vi "CPP-BLplotter.vi"(0 "Plot Array":cluster{dbl[], dbl[]}[](array[cluster]) {"?" format="%.2f"; "?" format="%.2f"}, 1 "Job Directory":path) -> (2 "Saved Automatically?":bool, 3 "gnuplotScript":string, 4 "Plot data file":path)   [LabVIEW 2014]
uses:
  gnuplotScriptComponents/BLPlottersubVIs/BLTarget.ctl
  gnuplotScriptComponents/BLPlottersubVIs/Resampler.ctl
  gnuplotScriptComponents/at.ctl
  Results_plotter_Global.vi
panel:
  in  "Tab Control":enum32{"Good Shit", "Targets", "Boring Shit"}(tab)
  in  "NormaliseHeight?":bool
  in  "oneshot":bool=TRUE
  in  "U(h)":dbl
  in  "Fit Zmin":dbl=100.0 min=0.0 max=200.0 step=20.0
  in  "autoprint":bool
  out "with d0":cluster{"n":dbl, "d0":dbl, "d0 2":dbl} {"d0 2" format="%#.1e"; "d0" format="%#.1f"; "n" format="%.3f"}
  in  "Fit Zmax":dbl=550.0 min=0.0 max=2000.0 step=50.0
  out "lambda-":dbl format="%_2g"
  out "lambda+":dbl format="%_2g"
  out "lambda(h)":dbl format="%.3g"
  in  "HeightJitter%":dbl min=0.0 max=20.0 step=1.0
  in  "Spectra Folder::":path
  out "Spectrum":cluster{"all rows":dbl[], "all rows":dbl[]}[](graph)
  in  "Stop Button":bool
  in  "Print Button":bool
  out "U,L(U)":cluster{dbl[], dbl[]}[](graph)
  out "TI,Sigma":cluster{dbl[], dbl[]}[](graph)
  in  "MaxFitFreq":dbl
  in  "lambdaSpan(%)":dbl
  in  "integralTweak":dbl=1.0 min=0.8 max=1.2 step=0.01
  out "case":string
  out "No d0":cluster{"n":dbl, "d0":dbl, "d0 2":dbl} {"d0 2" format="%#.1e"; "n" format="%.3f"}
  in  "Spectra?":bool
  in  "Scale":dbl=1.0 min=1.0 max=10000.0 step=50.0
  in  "Zref":dbl=508.0 min=0.0 step=25.0
  in  "BL Scratchpad":T1[](array[typedef]) {"n" min=0.02 max=0.5 step=0.01 format="%.2f"}
  in  "Boundary Layer Targets Folder":path=path "Data plotting/BLplotterExampleProfiles"
  out "BL Targets":T1[](array[typedef]) {"n" min=0.02 max=0.5 step=0.01 format="%.2f"}
  in  "OutputType":enum16{"PDF", "PNG-ReportStyle"}(ring)
  out "File Path Control":path
  in  "Resampler":T2
  in  "ResampleToN":i32=12
  in  "ResampleHeights":dbl[](array[numeric])=[25.4, 38.1, 50.8, 76.2, 101.6, 127.0, 152.4, 203.2, 254.0, 304.8, 406.4, 508.0, 609.6, 812.8, 1219.2, 1524.0]
  in  "Use for:":T3(array[ring])=[enum."\nU", enum."\nLambda", enum."\nTI", enum."\nSigma"]
  out "Incoming Titles":string[](array[string])
  in  "Plot Title":u16(ring) items=["Title String Only", "Roughness::", "TripSpire::", "Addl::", "Setup:wAddl:", "Spires::", "Trip:Height:(in)", "Trip:FromSpires:(in)", "AE::", "AE:n:", "AE:Pitch:(in)", "AE:Pitch:Pattern", "Date::", "Run:Start Time:", "Time:Stamp:", "Comments::", "Notes::", "XY::", "X:(mm):", "Y:(mm):", "Z:Floor:(mm)", "Z:Trav:(mm)", "\\overline{U}::/U_{ref}", "\\lambda(U):Est:(mm)", "TI(U)::(%)", "\\sigma(U)/U_{ref}::", "\\overline{u'w'}::", "\\overline{V}::/U_{ref}", "\\overline{W}::/U_{ref}", "\\overline{|UW|}/U_{ref}::", "TI(V)::(%)", "TI(W)::(%)", "TI_{UVW}::(%)", "\\sigma(V)/U_{ref}::", "\\sigma(W)/U_{ref}::", "u_*::", "U'/u_*::", "V'/u_*::", "W'/u_*::", "U_{Ref}::", "Decimation::", "AF:Reduction:(ms)", "\\overline{U}::", "\\overline{V}::", "\\overline{W}::", "\\overline{|UW|}::", "\\overline{UVW}::", "\\sigma^2(U)::", "\\sigma^2(V)::", "\\sigma^2(W)::", "\\sigma^2(|UW|)::", "\\sigma^2(UVW)::", "\\overline{u'v'}::", "\\overline{v'w'}::", "\\overline{\\theta}::", "\\sigma^2(\\theta)::", "AF:GoodOut:Valid", "AF:GoodP:Valid", "\\tau(U)::", "Reference:Temperature:Used for Corrections", "Atmos:Pressure:Used for Corrections", "X:(URef):(mm)", "Y:(URef):(mm)", "Z:(URef):(mm)", "Z1000byX::", "Tunnel1 Metadata:Z:Corrections", "Row:Type:", "Point:Time:", "Meas:Insts:", "Run:Messages:", "Original:Results:Filename", "Current:Data:Filename", "Current:Data File:1st Folder level", "Current:Data File:2nd Folder level", "Current:Data File:3rd Folder level", "Current:Data File:4th Folder level", "Current:File:Number", "Raw:Data:Filename", "AE:Density:", "AE:Fetch:(m)", "U:/U_{510}:", "Wind:Direction:deg", "U_{510}::", "n:ESDUHeights: Z 100.0 - 1050.0", "nd:ESDUHeights: Z 100.0 - 1050.0", "d0:ESDUHeights: Z 100.0 - 1050.0", "Flow:Measurement:Time", "Setup:TripMove:", "n:AsTaken: Z 40.0 - 500.0", "nd:AsTaken: Z 40.0 - 500.0", "d0:AsTaken: Z 40.0 - 500.0", "n:AsTaken: Z 55.0 - 500.0", "nd:AsTaken: Z 55.0 - 500.0", "d0:AsTaken: Z 55.0 - 500.0", "TI:at:254", "TI:at:508", "RMS(U)::", "Number of Measurements"]
  out "Final Title":string
  in  "Plot Title Post Block":string
  in  "Plot Title Pre Block":string="Test"
  in  "Show Script Editor?":bool
  in  "OpenLogfile?":bool
  out "spectraLegend":string[](array[string])
  in  "SpecificPlotFolder":string="DescriptiveFolderName"
  # "Fit using values at  measurement Z heights"
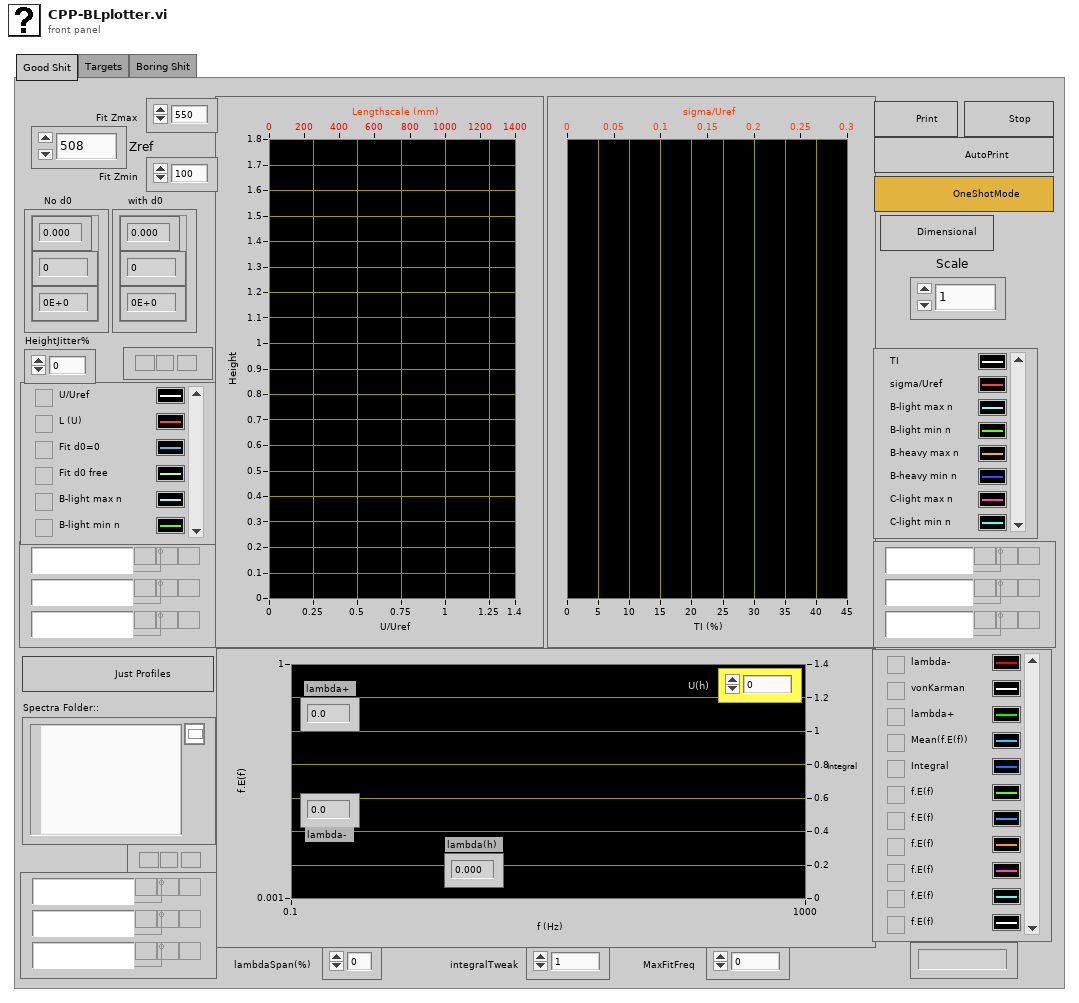
[diagram p1: front panel]
types:
  T1 = typedef "BLTarget.ctl" = cluster{"Code":string, "TI Profile (FS)":dbl[][], "n":dbl}
  T2 = typedef "Resampler.ctl" = enum32{"AsTaken", "Regular", "Prescribed"}
  T3 = enum16{"Don't Use", "\nU", "\nLambda", "\nTI", "\nSigma"}[]
  T4 = typedef "at.ctl" = cluster{"XcoordSys":string, "YcoordSys":string, "Xvalue":dbl, "Yvalue":dbl}
  T5 = typedef "LVRangeTypeDef.ctl" = cluster{"Minimum":dbl, "Maximum":dbl, "Increment":dbl, "Minor Increment":dbl, "Start":dbl}
  T6 = typedef "PowerLaw.ctl" = cluster{"n":dbl, "d0":dbl, "Residual":dbl}
  T7 = cluster{"TI Profile (FS)":dbl[], "Array":dbl[]}[]
  T8 = cluster{"Array":dbl[], "best nonlinear fit":dbl[]}
  T9 = cluster{"Plot.Plot Name":string, "Plot.Plot Color":u32, "Plot.Visible?":bool}
  T10 = typedef "minAndMax.ctl" = cluster{"Min":T11, "Max":T11}
  T11 = typedef "AutoManualNumber.ctl" = cluster{"Auto":bool, "Value":dbl}
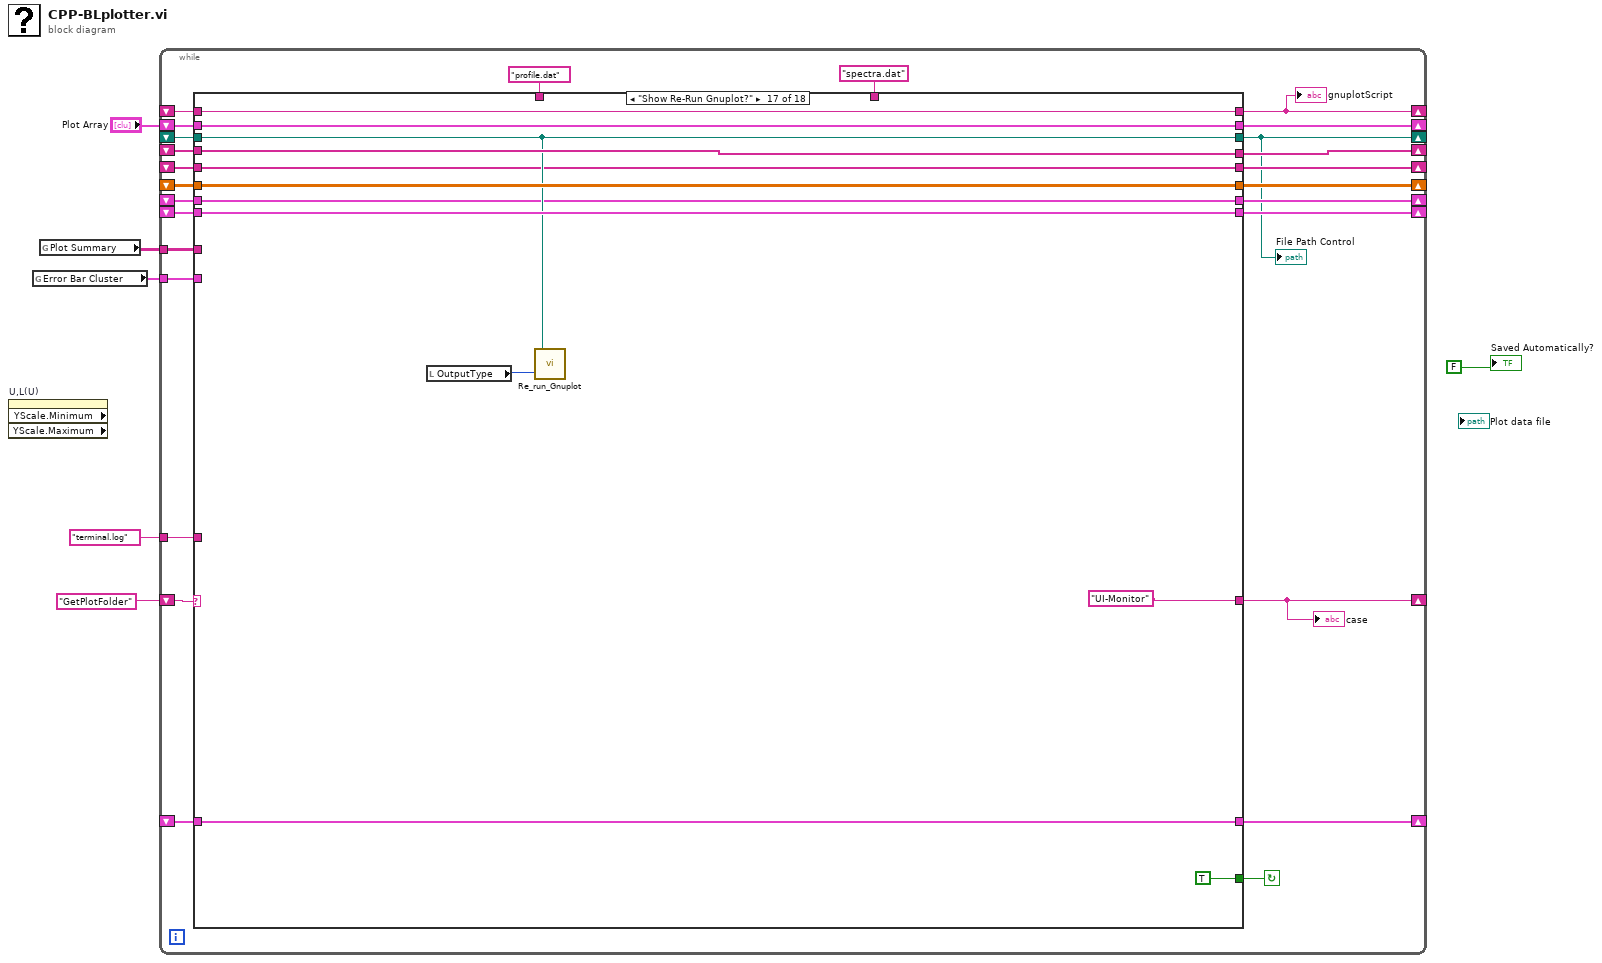
[diagram p0: block diagram]
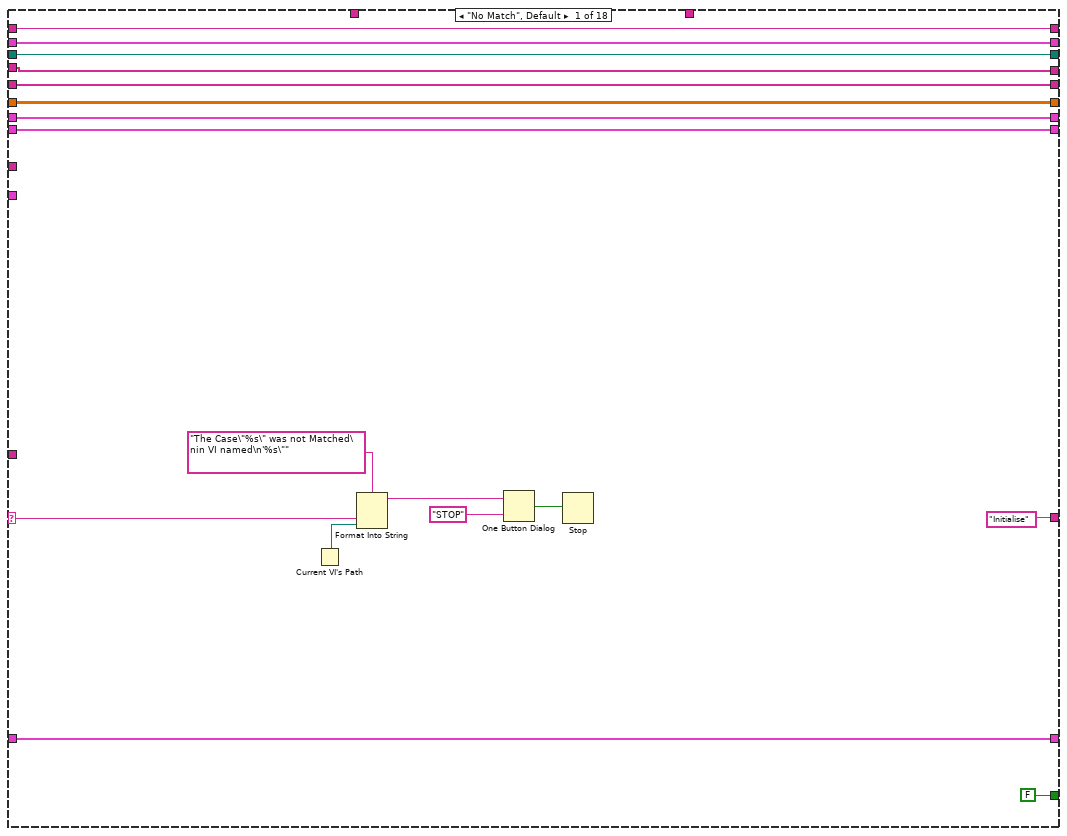
[diagram p2: hidden frame]
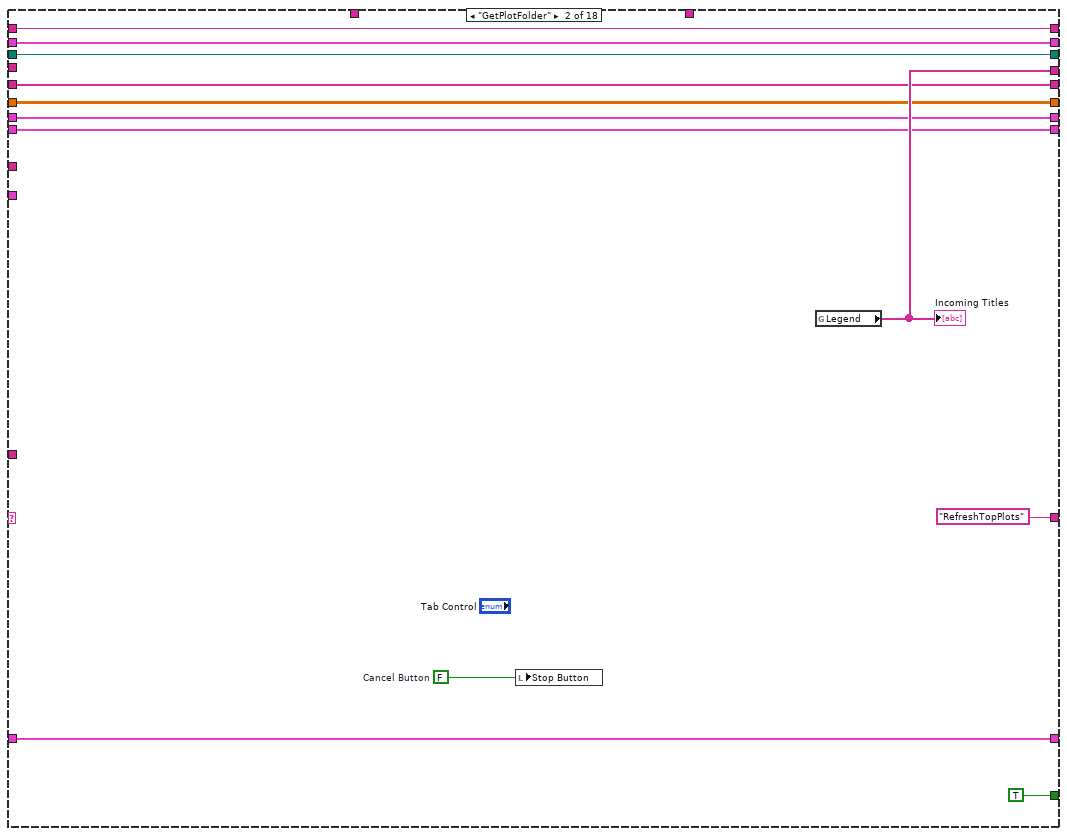
[diagram p3: hidden frame]
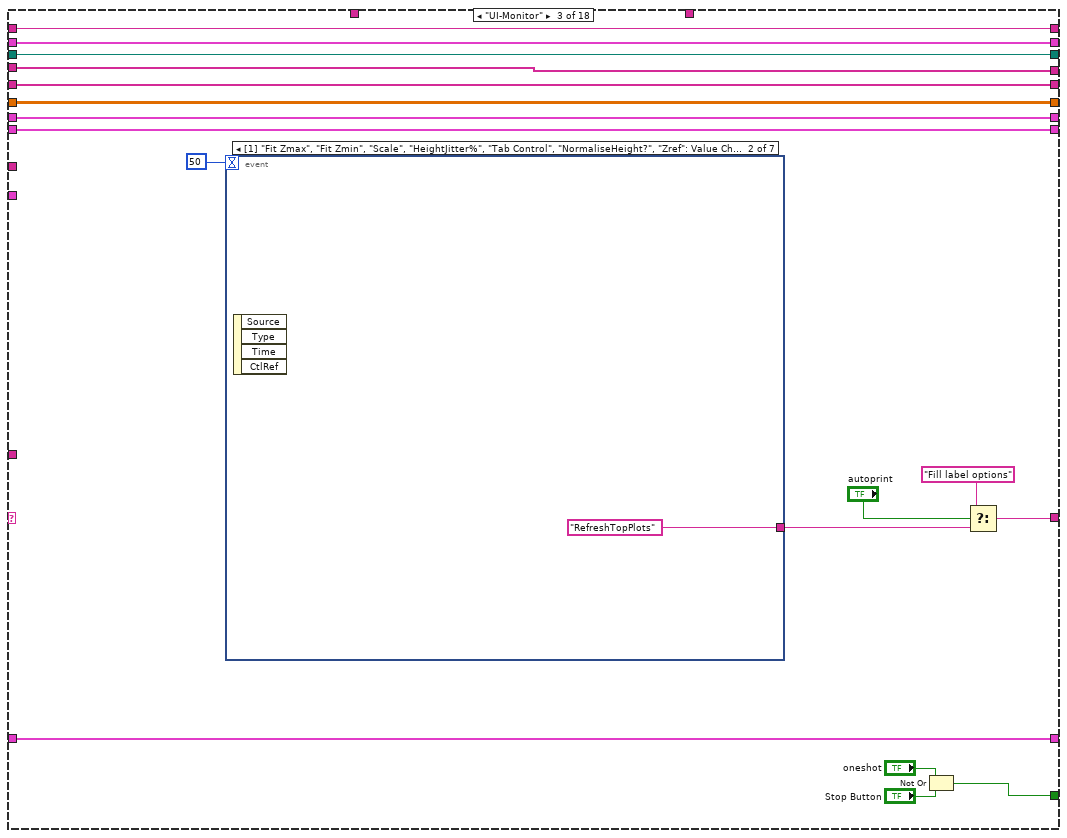
[diagram p4: hidden frame]
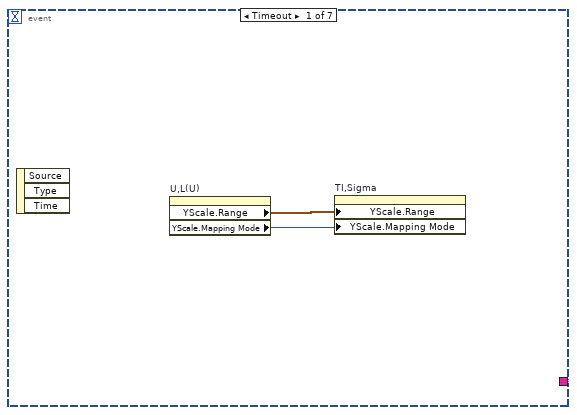
[diagram p5: hidden frame]
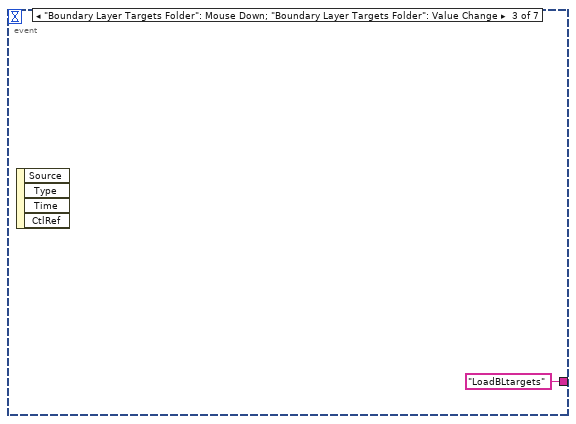
[diagram p6: hidden frame]
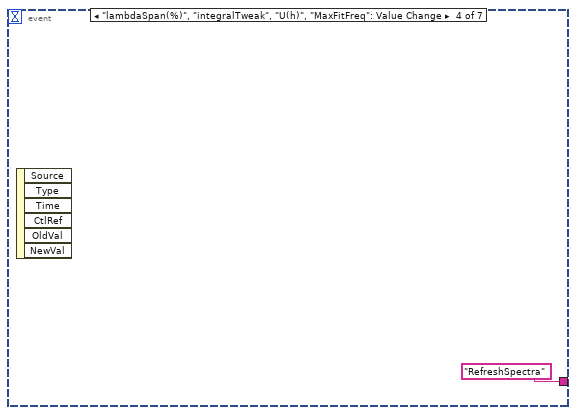
[diagram p7: hidden frame]
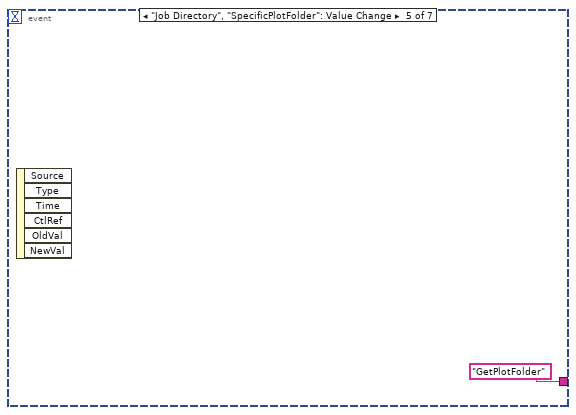
[diagram p8: hidden frame]
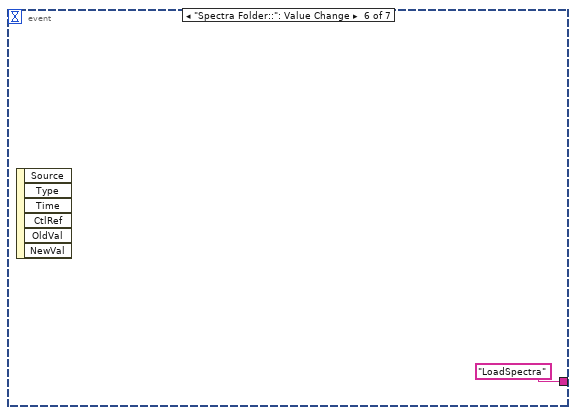
[diagram p9: hidden frame]
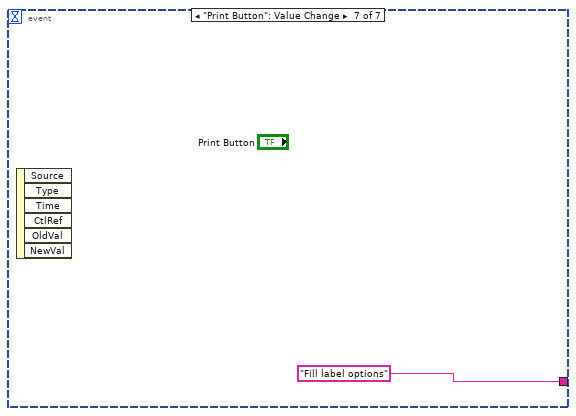
[diagram p10: hidden frame]
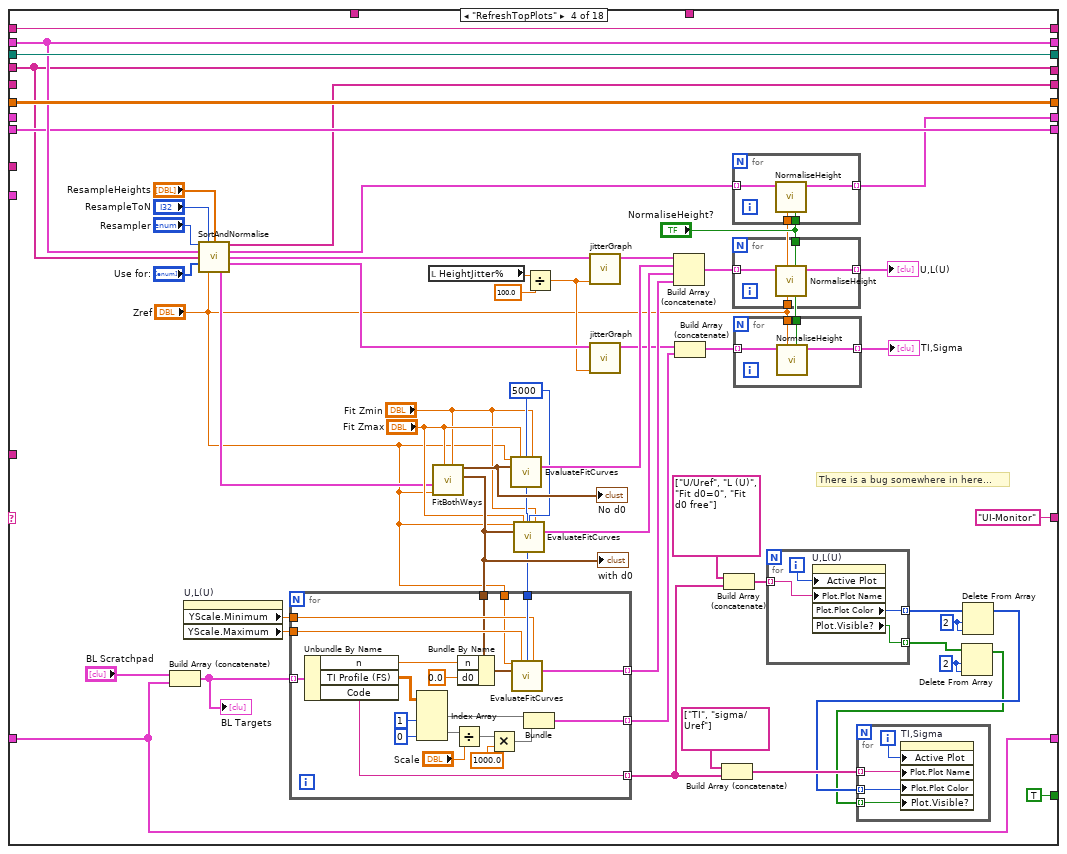
[diagram p11: hidden frame]
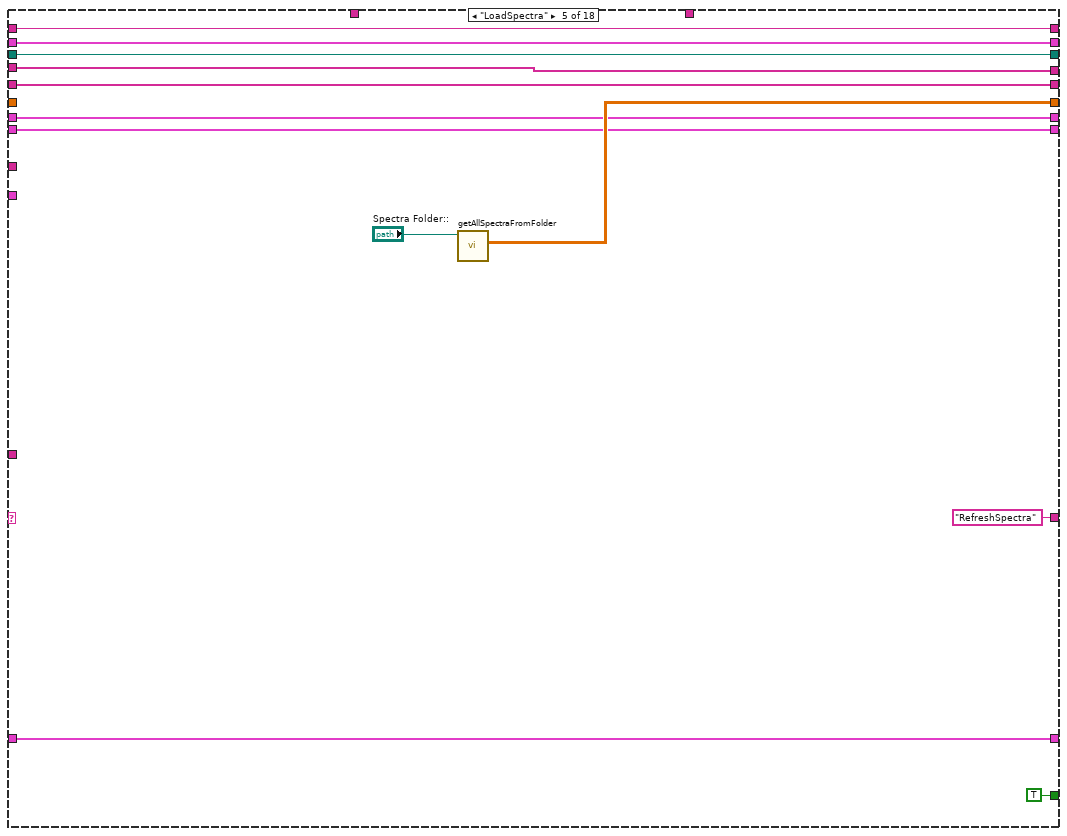
[diagram p12: hidden frame]
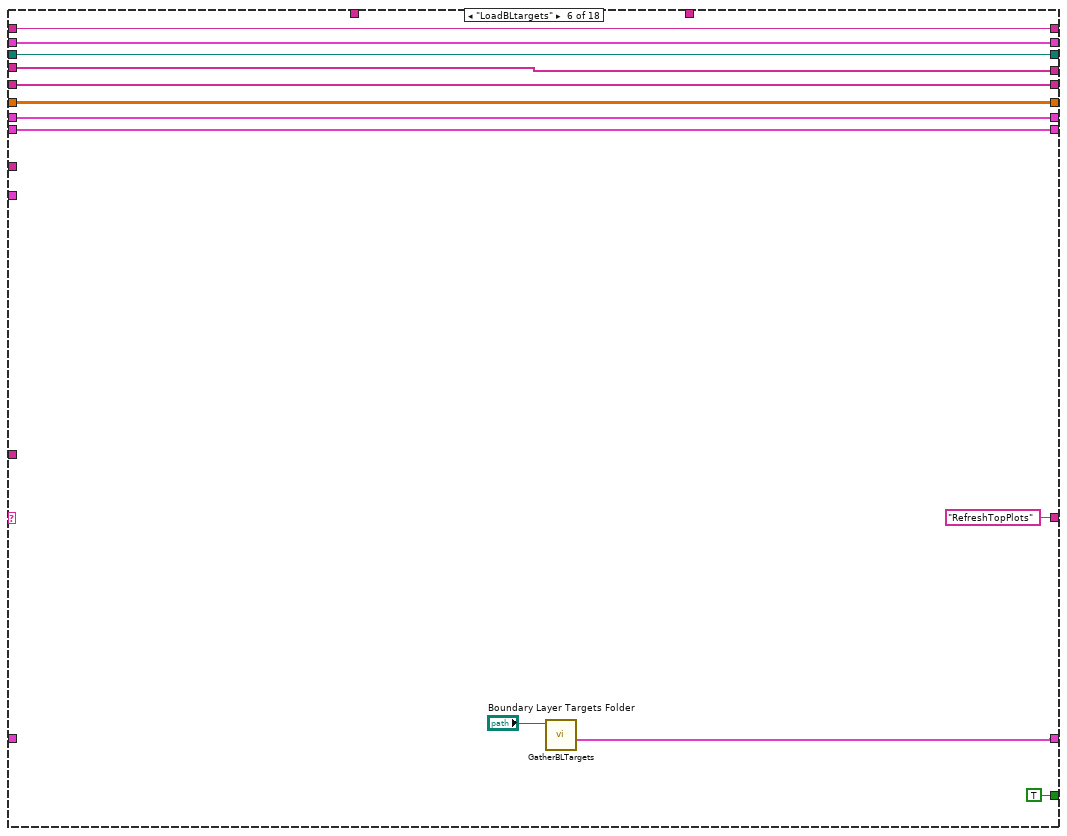
[diagram p13: hidden frame]
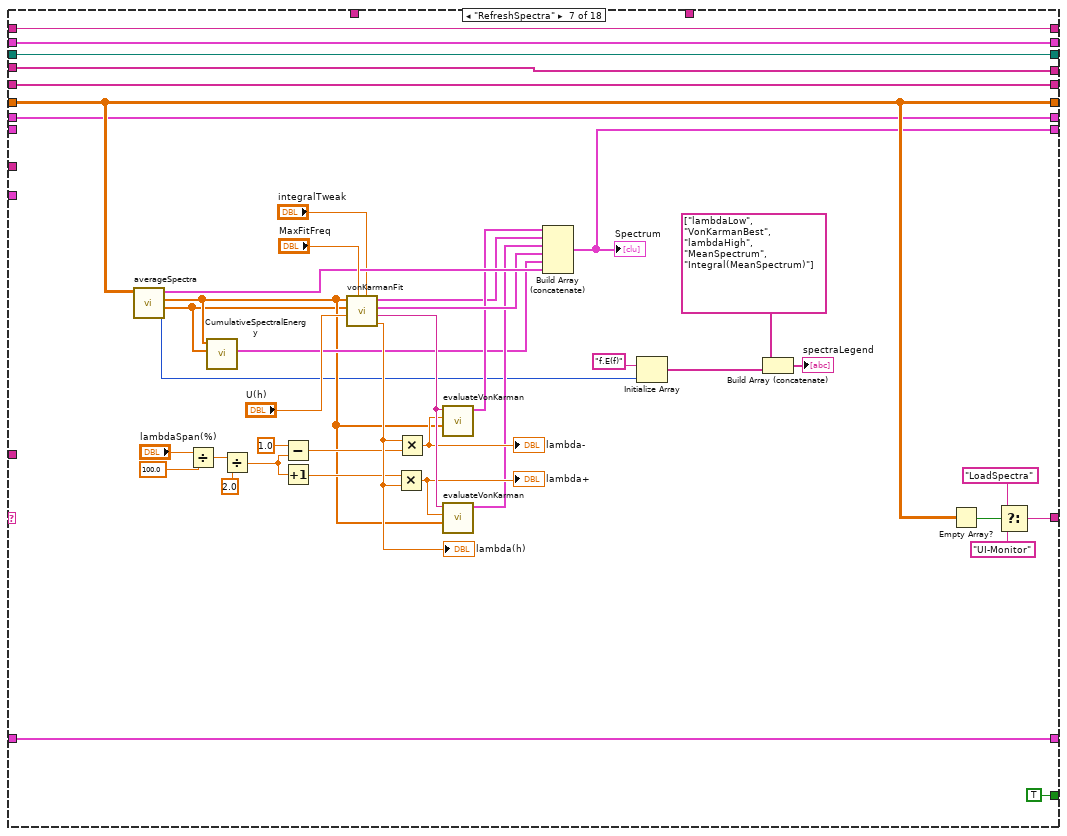
[diagram p14: hidden frame]
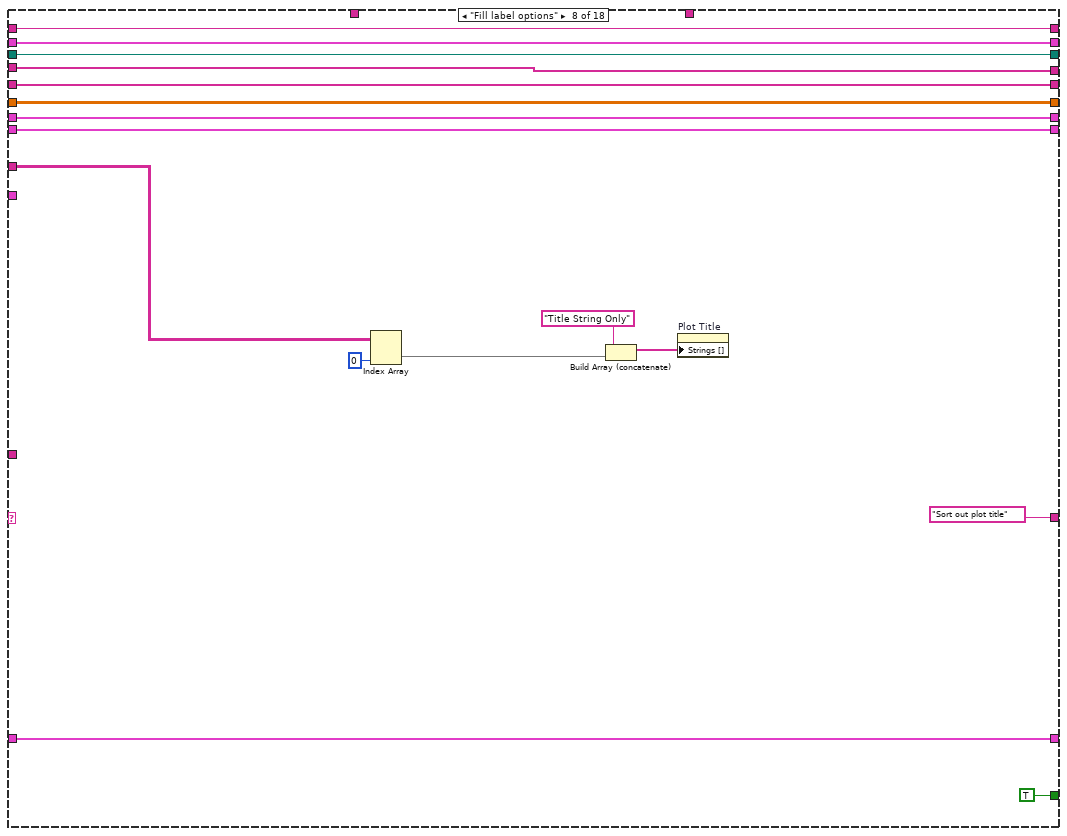
[diagram p15: hidden frame]
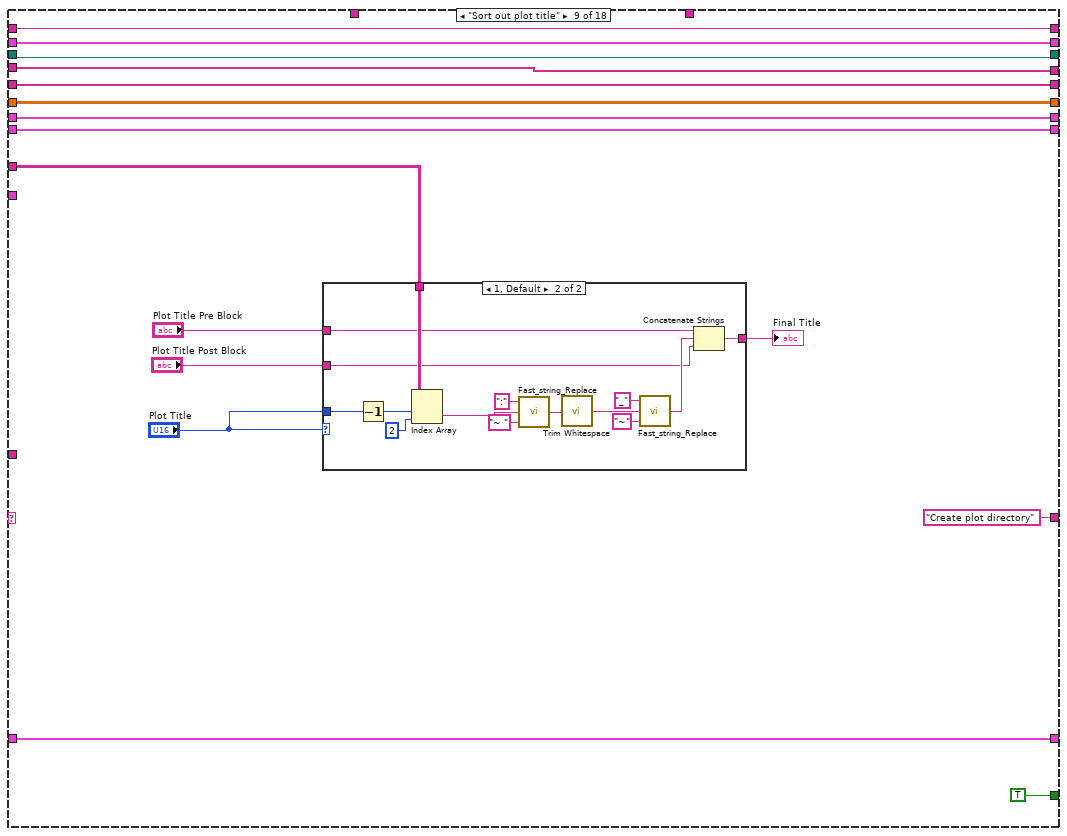
[diagram p16: hidden frame]
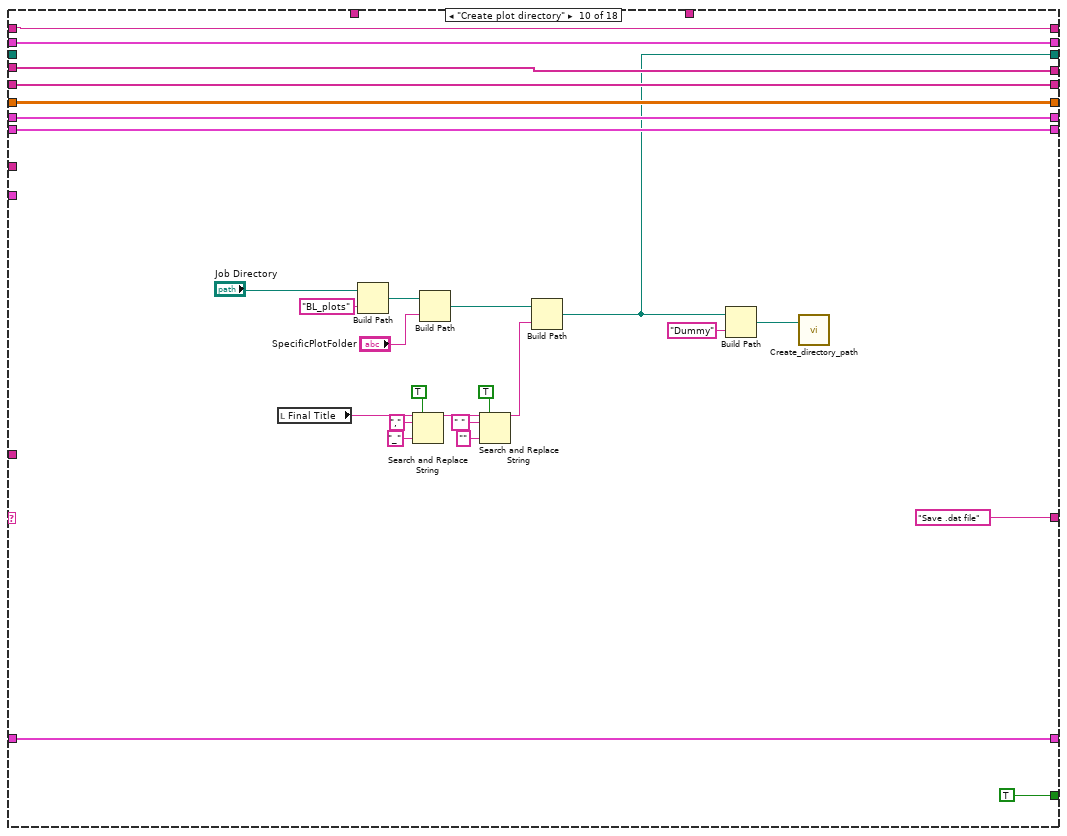
[diagram p18: hidden frame]
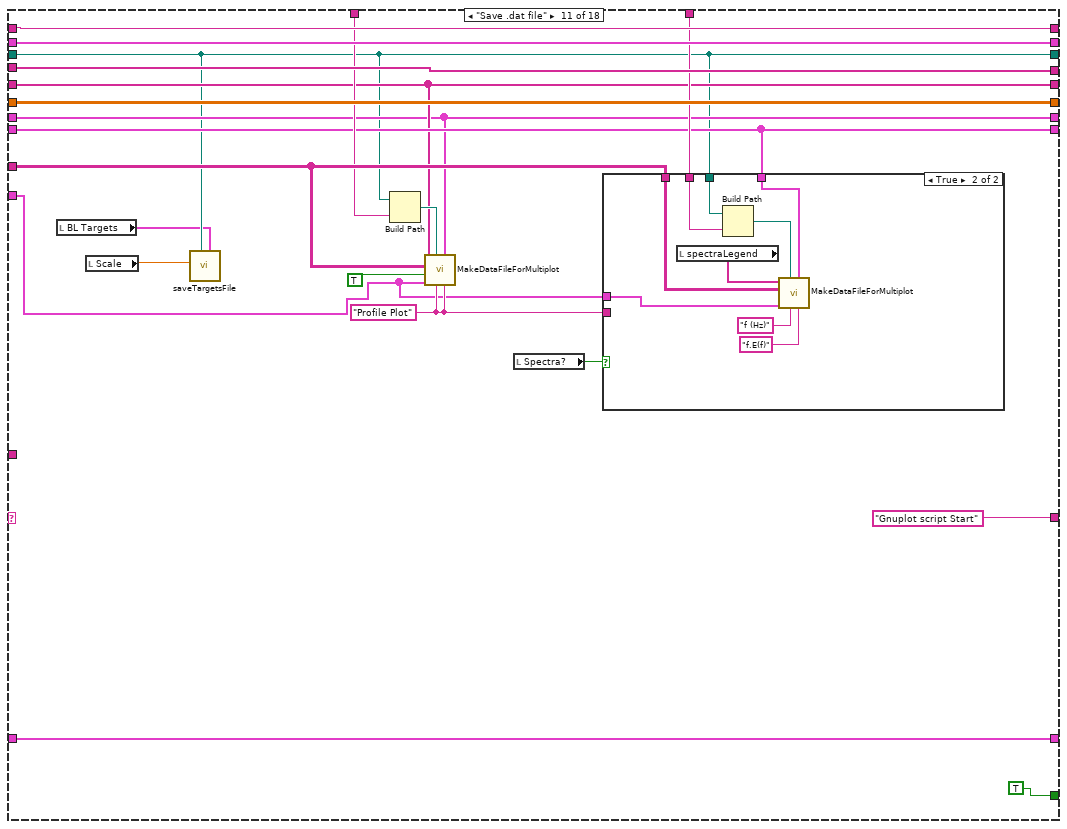
[diagram p19: hidden frame]
diagram:
  n1 = property on="U,L(U)" class="XYGraph (strict)" props=["YScale", "Minimum", "YScale", "Maximum"]() -> ()  [unwired: 2 in, 4 out]
  n2 = global read "Results_plotter_Global.vi" "Error Bar Cluster"() -> (w1:cluster{string[]}[])
  n3 = global read "Results_plotter_Global.vi" "Plot Summary"() -> (w5:string[][])
  n4 = while {
    shift-left: "GetPlotFolder" -> [w31]
    shift-right: [w24] -> _
    tunnel: w5 -> [w30]
    shift-right: [w9] -> _
    shift-left: _ -> [w29]
    shift-right: [w15] -> _
    shift-left: "Plot Array" -> [w28]
    shift-right: [w21] -> _
    shift-left: _ -> [w27]
    shift-right: [w13] -> _
    shift-left: _ -> [w26]
    tunnel: "terminal.log" -> [w25]
    shift-right: [w23] -> _
    shift-left: _ -> [w22]
    shift-right: [w20] -> _
    shift-left: _ -> [w19]
    shift-right: [w16] -> _
    shift-left: _ -> [w14]
    shift-right: [w12] -> _
    shift-left: _ -> [w11]
    tunnel: w1 -> [w10]
    shift-right: [w7] -> _
    shift-left: _ -> [w8]
    stop <- w32 continue-if-true
    n5 = case shown="\"Show Re-Run Gnuplot?\"" w31 {
      selector: w31 -> [w38 _ _ _ _ _ _ _ _ _ _ _ _ _ _ _ _ _]
      tunnel: [FALSE TRUE w63 TRUE ("Top Level") TRUE ("Top Level") TRUE ("Top Level") TRUE ("Top Level") TRUE ("Top Level") TRUE ("Top Level") TRUE TRUE ("Top Level") TRUE ("Top Level") TRUE ("Top Level") TRUE ("Top Level") TRUE ("Top Level") w504 TRUE ("Top Level") TRUE ("Top Level")] -> w32
      tunnel: ["Initialise" "RefreshTopPlots" w69 "UI-Monitor" ("t") "RefreshSpectra" ("t") "RefreshTopPlots" ("t") w221 "Sort out plot title" "Create plot directory" ("t") "Save .dat file" "Gnuplot script Start" w378 "Write gnuplot file" ("t") "Execute shell script" ("t") "Has pdf been generated?" ("t") w513 "UI-Monitor" ("t") "UI-Monitor" ("t")] -> w24
      tunnel: w30 -> [_ _ _ _ _ _ _ w264 w275 _ w338 _ _ _ _ _ _ _]
      tunnel: [w42 w51 w75 w141 w194 w206 w248 w259 w269 w312 w329 w383 w464 w472 w488 w516 w525 w535] -> w9
      tunnel: w29 -> [w42 w51 w75 w141 w194 w206 w248 w259 w269 _ w329 w383 w464 w472 w488 w516 w525 w535]
      tunnel: w28 -> [w41 w58 w76 w135 w193 w205 w247 w260 w280 w323 w340 w388 w463 w482 w501 w519 w531 w545]
      tunnel: [w41 w58 w76 w135 w193 w205 w247 w260 w280 w323 w340 w388 w463 w482 w501 w519 w531 w545] -> w15
      tunnel: w27 -> [w40 w59 w77 w140 w192 w204 w246 w261 w276 w322 w344 _ w449 w467 w499 w517 w529 w543]
      tunnel: [w40 w59 w77 w140 w192 w204 w246 w261 w276 w322 w344 w361 w453 w467 w499 w517 w529 w543] -> w21
      tunnel: [w39 w56 w74 w126 w191 w203 w245 w258 w279 w321 w341 w387 w462 w477 w500 w518 w530 w544] -> w13
      tunnel: w26 -> [w39 _ w74 w126 w191 w203 w245 w258 w279 w321 w341 w387 w462 w477 w500 w518 w530 w544]
      tunnel: w25 -> [_ _ _ _ _ _ _ _ _ _ _ _ _ _ w496 _ _ w539]
      tunnel: [w37 w55 w78 w139 w189 w197 w216 w254 w271 w318 w339 w385 w461 w474 w495 w509 w527 w537] -> w23
      tunnel: w22 -> [w37 w55 w78 w139 _ w197 w216 w254 w271 w318 w339 w385 w461 w474 w495 w509 w527 w537]
      tunnel: [w36 w54 w72 w128 w186 w200 w215 w253 w270 w317 w333 w384 w460 w473 w494 w508 w526 w536] -> w20
      tunnel: w19 -> [w36 w54 w72 w128 w186 w200 _ w253 w270 w317 w333 w384 w460 w473 w494 w508 w526 w536]
      tunnel: "profile.dat" ("name or relative path") -> [_ _ _ _ _ _ _ _ _ _ w337 w371 _ _ _ _ _ _]
      tunnel: "spectra.dat" ("name or relative path") -> [_ _ _ _ _ _ _ _ _ _ w336 _ w452 _ _ _ _ _]
      tunnel: [w35 w53 w71 w90 w185 w199 w209 w251 w267 w314 w331 w382 w459 w471 w493 w507 w524 w534] -> w16
      tunnel: w14 -> [w35 w53 w71 _ w185 w199 w209 w251 w267 w314 w331 w382 w459 w471 w493 w507 w524 w534]
      tunnel: [w34 w52 w70 w125 w184 w198 w208 w250 w266 w313 w332 w381 w458 w470 w492 w506 w523 w533] -> w12
      tunnel: w11 -> [w34 w52 w70 _ w184 w198 w208 w250 w266 w313 w332 w381 w458 w470 w492 w506 w523 w533]
      tunnel: w10 -> [_ _ _ _ _ _ _ _ _ _ w326 _ _ _ _ _ _ _]
      tunnel: w8 -> [w33 w50 w62 w97 w183 _ w207 w249 w265 w297 w324 w372 w433 w465 w484 w502 w521 w532]
      tunnel: [w33 w50 w62 w97 w183 w195 w207 w249 w265 w297 w324 w372 w433 w465 w484 w502 w521 w532] -> w7
      frame "No Match", Default {
        n6 = Current VI's Path() -> (path=w44:path)
        n7 = Format Into String(format string="The Case\"%s\" was not Matched\nin VI named\n'%s\"" ("Format String"), w38, w44) -> (resulting string=w47:string)  [unwired: 2 in, 1 out]
        n8 = One Button Dialog(message=w47, button name ("OK")="STOP") -> (true=w45:bool)
        n9 = Stop(stop? (T)=w45) -> ()
      }
      frame "GetPlotFolder" {
        w57 = FALSE  # Cancel Button
        n10 = local write "Stop Button"(w57) -> ()
        n11 = global read "Results_plotter_Global.vi" "Legend"() -> (w56:string[])
        "Incoming Titles" <- w56
      }
      frame "UI-Monitor" {
        n12 = event shown="[1] \"Fit Zmax\", \"Fit Zmin\", \"Scale\", \"HeightJitter%\", \"Tab Control\", \"NormaliseHeight?\", \"Zref\": Value Change;  \"U,L(U)\": Plot Attribute Change" {
          selector: _ -> [_ _ _ _ _ _ _]
          dyn-events: _ -> [_ _ _ _ _ _ _]
          timeout: 50 -> [_ _ _ _ _ _ _]
          tunnel: ["UI-Monitor" "RefreshTopPlots" "LoadBLtargets" "RefreshSpectra" "GetPlotFolder" "LoadSpectra" "Fill label options"] -> w66
          event Timeout {
            n13 = event-data() -> ()  [unwired: 1 in, 3 out]
            n14 = property on="U,L(U)" class="XYGraph (strict)"() -> ("YScale.Range"=w79:T5, "YScale.Mapping Mode"=w80:u8)  [unwired: 2 in, 2 out]
            n15 = property on="TI,Sigma" class="XYGraph (strict)"("YScale.Range"=w79, "YScale.Mapping Mode"=w80) -> ()  [unwired: 2 in, 2 out]
          }
          event "Fit Zmax", "Fit Zmin", "Scale", "HeightJitter%", "Tab Control", "NormaliseHeight?", "Zref": Value Change; "U,L(U)": Plot Attribute Change {
            n16 = event-data() -> ()  [unwired: 1 in, 4 out]
          }
          event "Boundary Layer Targets Folder": Mouse Down; "Boundary Layer Targets Folder": Value Change {
            n17 = event-data() -> ()  [unwired: 1 in, 4 out]
          }
          event "lambdaSpan(%)", "integralTweak", "U(h)", "MaxFitFreq": Value Change {
            n18 = event-data() -> ()  [unwired: 1 in, 6 out]
          }
          event "Job Directory", "SpecificPlotFolder": Value Change {
            n19 = event-data() -> ()  [unwired: 1 in, 6 out]
          }
          event "Spectra Folder::": Value Change {
            n20 = event-data() -> ()  [unwired: 1 in, 6 out]
          }
          event "Print Button": Value Change {
            n21 = event-data() -> ()  [unwired: 1 in, 6 out]
          }
        }
        n22 = Not Or(1:"Stop Button", 2:"oneshot") -> (0:w63:bool)
        n23 = Select(t="Fill label options", s="autoprint", f=w66) -> (s? t:f=w69:string)
      }
      frame "RefreshTopPlots" {
        w105 = 2 ("length")
        w106 = 2 ("length")
        w118 = 5000
        # "There is a bug somewhere in here..."
        n24 = Build Array (concatenate)("BL Scratchpad", w97) -> (w102:T1[])
        "BL Targets" <- w102
        n25 = property on="U,L(U)" class="XYGraph (strict)"() -> ("YScale.Minimum"=w123:dbl, "YScale.Maximum"=w122:dbl)  [unwired: 2 in, 2 out]
        n26 = call "SortAndNormalise.vi"("Resampler"="Resampler", "ResampleToN"="ResampleToN", "ResampleHeights"="ResampleHeights", "Plot Array In"=w135, "LegendsIn"=w126, "Use for:"="Use for:", "Zref"="Zref") -> ("SortedLegends"=w125:string[], "SortedData"=w91:cluster{"Array":dbl[], "Array":dbl[]}[], "LeftGraph"=w132:cluster{"Array":dbl[], "Array":dbl[]}[], "RightGraph"=w130:cluster{"Array":dbl[], "Array":dbl[]}[], "UzClusterOutput"=w96:cluster{"Array":dbl[], "Array":dbl[]})  [unwired: 4 in]
        n27 = local read "HeightJitter%"() -> (w137:dbl)
        n28 = call "FitBothWays.vi"("Fit Zmin"="Fit Zmin", "Fit Zmax"="Fit Zmax", "Zref"="Zref", "zUCluster in"=w96) -> ("PowerLawWithDisplacement"=w120:T6, "PowerLawNoDisplacement"=w121:T6)  [unwired: 6 in]
        "No d0" <- w121
        "with d0" <- w120
        n29 = for {
          tunnel: [w182] -> w119 mode=indexing
          tunnel: w118 -> [w181]
          tunnel: w123 -> [w180]
          tunnel: w122 -> [w179]
          tunnel: w102 -> [w178] mode=indexing
          tunnel: w120 -> [w176]
          tunnel: [w173] -> w115 mode=indexing
          tunnel: [w163] -> w114 mode=indexing
          tunnel: "Zref" -> [w162]
          n30 = Unbundle By Name(w178) -> ("n"=w175:dbl, "TI Profile (FS)"=w164:dbl[][], "Code"=w163:string)
          n31 = Index Array(array=w164, index (col) #1=1 ("disabled index (col)"), index (col) #2=0 ("index (col)")) -> (element #1=w170:dbl[], element #2=w168:dbl[])  [unwired: 2 in]
          n32 = Divide(x=w168, y="Scale") -> (x/y=w169:dbl[])
          n33 = Bundle By Name(cluster=w176, "n"=w175, "d0"=0.0) -> (w177:T6)
          n34 = Multiply(x=w169, y=1000.0) -> (x*y=w166:dbl[])
          n35 = call "EvaluateFitCurves.vi"("Zref"=w162, "Fit Zmax"=w179, "nPoints"=w181, "Fit Zmin"=w180, "PowerLaw"=w177) -> ("PlotCluster"=w182:cluster{"Array":dbl[], "Array":dbl[]})  [unwired: 10 in]
          n36 = Bundle("TI Profile (FS)"=w170, w166) -> (w173:cluster{"TI Profile (FS)":dbl[], dbl[]})  [unwired: 1 in]
        }
        n37 = call "EvaluateFitCurves.vi"("Zref"="Zref", "Fit Zmax"="Fit Zmax", "nPoints"=w118, "Fit Zmin"="Fit Zmin", "PowerLaw"=w121) -> ("PlotCluster"=w127:cluster{"Array":dbl[], "Array":dbl[]})  [unwired: 10 in]
        n38 = call "EvaluateFitCurves.vi"("Zref"="Zref", "Fit Zmax"="Fit Zmax", "nPoints"=w118, "Fit Zmin"="Fit Zmin", "PowerLaw"=w120) -> ("PlotCluster"=w124:cluster{"Array":dbl[], "Array":dbl[]})  [unwired: 10 in]
        n39 = Divide(x=w137, y=100.0) -> (x/y=w129:dbl)
        n40 = call "jitterGraph.vi"("Y-jitter"=w129, "GraphPlots"=w132) -> ("jitteredGraphPlots"=w131:cluster{"Array":dbl[], "Array":dbl[]}[])  [unwired: 9 in]
        n41 = call "jitterGraph.vi"("Y-jitter"=w129, "GraphPlots"=w130) -> ("jitteredGraphPlots"=w116:cluster{"Array":dbl[], "Array":dbl[]}[])  [unwired: 9 in]
        n42 = Build Array (concatenate)(w131, w127, w124, w119) -> (w95:cluster{"Array":dbl[], "Array":dbl[]}[])
        n43 = Build Array (concatenate)(w116, w115) -> (w93:T7)
        n44 = Build Array (concatenate)(string[] ["TI", "sigma/Uref"], w114) -> (w117:string[])
        n45 = Build Array (concatenate)(string[] ["U/Uref", "L (U)", "Fit d0=0", "Fit d0 free"], w114) -> (w109:string[])
        n46 = for {
          tunnel: w91 -> [w145] mode=indexing
          tunnel: [w144] -> w90 mode=indexing
          tunnel: "Zref" -> [w143]
          tunnel: "NormaliseHeight?" -> [w142]
          n47 = call "NormaliseHeight.vi"("NormaliseHeight?"=w142, "Zref"=w143, "Value-Z Cluster In"=w145) -> ("Value-Z Cluster Out"=w144:cluster{"Array":dbl[], "Array":dbl[]})  [unwired: 8 in]
        }
        n48 = for {
          tunnel: w95 -> [w153] mode=indexing
          tunnel: [w152] -> w94 mode=indexing
          tunnel: "NormaliseHeight?" -> [w151]
          tunnel: "Zref" -> [w150]
          n49 = call "NormaliseHeight.vi"("NormaliseHeight?"=w151, "Zref"=w150, "Value-Z Cluster In"=w153) -> ("Value-Z Cluster Out"=w152:cluster{"Array":dbl[], "Array":dbl[]})  [unwired: 8 in]
        }
        "U,L(U)" <- w94
        n50 = for {
          tunnel: w93 -> [w149] mode=indexing
          tunnel: [w148] -> w92 mode=indexing
          tunnel: "NormaliseHeight?" -> [w147]
          tunnel: "Zref" -> [w146]
          n51 = call "NormaliseHeight.vi"("NormaliseHeight?"=w147, "Zref"=w146, "Value-Z Cluster In"=w149) -> ("Value-Z Cluster Out"=w148:cluster{"Array":dbl[], "Array":dbl[]})  [unwired: 8 in]
        }
        "TI,Sigma" <- w92
        n52 = for {
          tunnel: w109 -> [w158] mode=indexing
          tunnel: [w161] -> w108 mode=indexing
          tunnel: [w160] -> w104 mode=indexing
          i -> [w159]
          n53 = property on="U,L(U)" class="XYGraph (strict)"("Active Plot"=w159, "Plot.Plot Name"=w158) -> ("Plot.Plot Color"=w161:u32, "Plot.Visible?"=w160:bool)  [unwired: 2 in, 2 out]
        }
        n54 = Delete From Array(array=w104, length=w105, index=w105) -> (array with subset deleted=w103:bool[])  [unwired: 1 out]
        n55 = Delete From Array(array=w108, length=w106, index=w106) -> (array with subset deleted=w107:u32[])  [unwired: 1 out]
        n56 = for {
          tunnel: w117 -> [w154] mode=indexing
          tunnel: w107 -> [w157] mode=indexing
          tunnel: w103 -> [w156] mode=indexing
          i -> [w155]
          n57 = property on="TI,Sigma" class="XYGraph (strict)"("Active Plot"=w155, "Plot.Plot Name"=w154, "Plot.Plot Color"=w157, "Plot.Visible?"=w156) -> ()  [unwired: 2 in, 2 out]
        }
      }
      frame "LoadSpectra" {
        n58 = call "getAllSpectraFromFolder.vi"("Spectra Folder::"="Spectra Folder::") -> ("spectra"=w189:dbl[][][])  [unwired: 10 in]
      }
      frame "LoadBLtargets" {
        n59 = call "GatherBLTargets.vi"("BL files folder path"="Boundary Layer Targets Folder") -> ("BL Targets out"=w195:T1[])  [unwired: 10 in]
      }
      frame "RefreshSpectra" {
        n60 = call "averageSpectra.vi"("multipleSpectra"=w216) -> ("nSpectra"=w213:i32, "meanSpectrum"=w217:dbl[], "frequencies"=w218:dbl[], "spectraPlots"=w242:cluster{"Array":dbl[], "Array":dbl[]}[])  [unwired: 7 in]
        n61 = Divide(x="lambdaSpan(%)", y=100.0) -> (x/y=w234:dbl)
        n62 = call "CumulativeSpectralEnergy.vi"("f.E(f)"=w217, "f"=w218) -> ("plottableBundle"=w225:cluster{"X":dbl[], "Array":dbl[]})  [unwired: 8 in, 1 out]
        n63 = Divide(x=w234, y=2.0 ("x")) -> (x/y=w227:dbl)
        n64 = Subtract(x=1.0, y=w227) -> (x-y=w236:dbl)
        n65 = Increment(x=w227) -> (x+1=w235:dbl)
        n66 = call "vonKarmanFit.vi"("integralTweak"="integralTweak", "MaxFitFreq"="MaxFitFreq", "U(h)"="U(h)", "f.E(f)"=w217, "f"=w218) -> ("lambda"=w237:dbl, "vonKarmanFitEquation"=w240:string, "CroppedData"=w241:cluster{"X Out":dbl[], "Y Out":dbl[]}, "FitCurve"=w229:T8)  [unwired: 3 in]
        "lambda(h)" <- w237
        n67 = Multiply(x=w235, y=w237) -> (x*y=w230:dbl)
        "lambda+" <- w230
        n68 = Multiply(x=w237, y=w236) -> (x*y=w231:dbl)
        "lambda-" <- w231
        n69 = call "evaluateVonKarman.vi"("frequencies"=w218, "lambda"=w231, "vonKarmanFitEquation"=w240) -> ("Cluster"=w232:cluster{"frequencies":dbl[], "Y Values":dbl[]})  [unwired: 8 in]
        n70 = call "evaluateVonKarman.vi"("frequencies"=w218, "lambda"=w230, "vonKarmanFitEquation"=w240) -> ("Cluster"=w228:cluster{"frequencies":dbl[], "Y Values":dbl[]})  [unwired: 8 in]
        n71 = Build Array (concatenate)(w232, w229, w228, w241, w225, w242) -> (w215:cluster{"Array":dbl[], "Array":dbl[]}[])
        "Spectrum" <- w215
        n72 = Initialize Array("f.E(f)", w213) -> (w212:string[])
        n73 = Build Array (concatenate)(string[] ["lambdaLow", "VonKarmanBest", "lambdaHigh", "MeanSpectrum", "Integral(MeanSpectrum)"], w212) -> (→"spectraLegend":string[])
        n74 = Empty Array?(array=w216) -> (empty?=w220:bool)
        n75 = Select(t="LoadSpectra", s=w220, f="UI-Monitor" ("t")) -> (s? t:f=w221:string)
      }
      frame "Fill label options" {
        n76 = Index Array(array=w264, index (col)=0 ("disabled index (col)")) -> (element=w256:string[])  [unwired: 1 in]
        n77 = Build Array (concatenate)("Title String Only", w256) -> (w255:string[])
        n78 = property on="Plot Title" class="Ring (strict)"("Strings []"=w255) -> ()  [unwired: 2 in, 2 out]
      }
      frame "Sort out plot title" {
        n79 = case shown="1, Default" "Plot Title" {
          tunnel: [w281 w286] -> w274
          tunnel: "Plot Title Pre Block" -> [w281 w285]
          tunnel: w275 -> [_ w289]
          tunnel: "Plot Title" -> [_ w288]
          tunnel: "Plot Title Post Block" -> [_ w282]
          frame 0 {
          }
          frame 1, Default {
            n80 = Decrement(x=w288) -> (x-1=w287:u16)
            n81 = Index Array(array=w289, index (row)=w287, index (col)=u16 2 ("y")) -> (element=w292:string)
            n82 = call "Fast_string_Replace.vi"("Replace match with:"="~ ", "Input String"=w292, "regular expression"=":") -> ("Output String"=w291:string)  [unwired: 2 out]
            n83 = call <vilib>:"Trim Whitespace.vi"("string"=w291) -> ("trimmed string"=w290:string)  [unwired: 1 in]
            n84 = call "Fast_string_Replace.vi"("Replace match with:"="~", "Input String"=w290, "regular expression"="_") -> ("Output String"=w284:string)  [unwired: 2 out]
            n85 = Concatenate Strings(w285, w284, w282) -> (w286:string)
          }
        }
        "Final Title" <- w274
      }
      frame "Create plot directory" {
        n86 = local read "Final Title"() -> (w311:string)
        n87 = Build Path(base path="Job Directory", name or relative path="BL_plots") -> (appended path=w298:path)
        n88 = Search and Replace String(replace all?=TRUE ("replace all? (F)"), input string=w311, search string=",", replace string="_" ("replace string (\"\")")) -> (result string=w304:string)  [unwired: 4 in, 3 out]
        n89 = Build Path(base path=w298, name or relative path="SpecificPlotFolder") -> (appended path=w301:path)
        n90 = Search and Replace String(replace all?=TRUE ("replace all? (F)"), input string=w304, search string=" ", replace string="" ("replace string (\"\")")) -> (result string=w303:string)  [unwired: 4 in, 3 out]
        n91 = Build Path(base path=w301, name or relative path=w303) -> (appended path=w312:path)
        n92 = Build Path(base path=w312, name or relative path="Dummy") -> (appended path=w316:path)
        n93 = call "Create_directory_path.vi"("Path name"=w316) -> ()  [unwired: 1 in, 2 out]
      }
      frame "Save .dat file" {
        w330 = "Profile Plot" ("X Axis Name")
        n94 = local read "BL Targets"() -> (w328:T1[])
        n95 = local read "Scale"() -> (w327:dbl)
        n96 = call "saveTargetsFile.vi"("BL Targets"=w328, "Path"=w329, "Scale"=w327) -> ()  [unwired: 9 in]
        n97 = Build Path(base path=w329, name or relative path=w337) -> (appended path=w334:path)
        n98 = call "MakeDataFileForMultiplot.vi"("Y Axis Name"=w330, "Plot Array"=w331, "X Axis Name"=w330, "Path"=w334, "Error Bar Cluster"=w326, "Transpose"=TRUE, "Plot Summary"=w338, "Legend"=w332) -> ()  [unwired: 4 in]
        n99 = local read "Spectra?"() -> (w325:bool)
        n100 = case shown="True" w325 {
          tunnel: w338 -> [_ w353]
          tunnel: w336 -> [_ w352]
          tunnel: w333 -> [_ w351]
          tunnel: w330 -> [_ _]
          tunnel: w329 -> [_ w350]
          tunnel: w326 -> [_ w349]
          frame False {
          }
          frame True {
            n101 = local read "spectraLegend"() -> (w345:string[])
            n102 = Build Path(base path=w350, name or relative path=w352) -> (appended path=w346:path)
            n103 = call "MakeDataFileForMultiplot.vi"("Y Axis Name"="f.E(f)", "Plot Array"=w351, "X Axis Name"="f (Hz)", "Path"=w346, "Error Bar Cluster"=w349, "Plot Summary"=w353, "Legend"=w345) -> ()  [unwired: 5 in]
          }
        }
      }
      frame "Gnuplot script Start" {
        # "Number of \"permanent\" plots"
        # "Number of \"permanent\" plots"
        n104 = local read "BL Targets"() -> (w357:T1[])
        n105 = Array Size(array=w357) -> (size(s)=w373:i32)
        n106 = Add(x=w373, y=4 ("x")) -> (x+y=w376:i32)
        n107 = for {
          N: w376 -> [_]
          tunnel: [w429] -> w356 mode=indexing
          i -> [w428]
          n108 = property on="U,L(U)" class="XYGraph (strict)"("Active Plot"=w428) -> ("Plot.Plot Name"=w432:string, "Plot.Plot Color"=w431:u32, "Plot.Visible?"=w430:bool)  [unwired: 2 in, 2 out]
          n109 = Bundle("Plot.Plot Name"=w432, "Plot.Plot Color"=w431, "Plot.Visible?"=w430) -> (w429:T9)  [unwired: 1 in]
        }
        n110 = local read "NormaliseHeight?"() -> (w368:bool)
        n111 = Add(x=w373, y=2 ("x")) -> (x+y=w374:i32)
        n112 = for {
          N: w374 -> [_]
          tunnel: [w425] -> w355 mode=indexing
          i -> [w423]
          n113 = property on="TI,Sigma" class="XYGraph (strict)"("Active Plot"=w423) -> ("Plot.Plot Name"=w424:string, "Plot.Plot Color"=w427:u32, "Plot.Visible?"=w426:bool)  [unwired: 2 in, 2 out]
          n114 = Bundle("Plot.Plot Name"=w424, "Plot.Plot Color"=w427, "Plot.Visible?"=w426) -> (w425:T9)  [unwired: 1 in]
        }
        n115 = local read "Final Title"() -> (w370:string)
        n116 = local read "Fit Zmax"() -> (w366:dbl)
        n117 = control-ref of="TI,Sigma"() -> (w358:refnum<vi>)
        n118 = control-ref of="U,L(U)"() -> (w359:refnum<vi>)
        n119 = local read "Fit Zmin"() -> (w365:dbl)
        n120 = local read "with d0"() -> (w362:cluster{"n":dbl, "d0":dbl, "d0 2":dbl})
        n121 = local read "No d0"() -> (w363:cluster{"n":dbl, "d0":dbl, "d0 2":dbl})
        n122 = local read "Scale"() -> (w360:dbl)
        n123 = local read "Zref"() -> (w367:dbl)
        n124 = case shown="\"PNG-ReportStyle\"" "OutputType" {
          tunnel: w371 -> [w405 w422]
          tunnel: w370 -> [w404 w421]
          tunnel: "Spectra?" -> [w403 w420]
          tunnel: w368 -> [w402 w419]
          tunnel: w367 -> [w401 w418]
          tunnel: w366 -> [w400 w417]
          tunnel: w365 -> [w399 w416]
          tunnel: "HeightJitter%" -> [w398 w415]
          tunnel: w363 -> [w397 w414]
          tunnel: w362 -> [w396 w413]
          tunnel: [w395 w412] -> w361
          tunnel: w360 -> [w394 w411]
          tunnel: w359 -> [w393 w410]
          tunnel: w358 -> [w392 w409]
          tunnel: w357 -> [w391 w408]
          tunnel: w356 -> [w390 w407]
          tunnel: w355 -> [w389 w406]
          frame "PDF", Default {
            n125 = call "AssembleBLMultiplotScript-UandTI.vi"("name or relative path"=w405, "Final Title"=w404, "Spectra?"=w403, "NormaliseHeight?"=w402, "Zref"=w401, "Fit Zmax"=w400, "Fit Zmin"=w399, "HeightJitter%"=w398, "Scale"=w394, "BL Targets"=w391, "U,L(U)"=w393, "UtargetsInfo"=w390, "TI,Sigma"=w392, "TItargetsInfo"=w389, "No d0"=w397, "with d0"=w396) -> ("gnuplotOut"=w395:string)  [unwired: 11 in]
          }
          frame "PNG-ReportStyle" {
            n126 = call "AssembleBLMultiplotScript-UandTI-CPPPNG.vi"("name or relative path"=w422, "Final Title"=w421, "Spectra?"=w420, "NormaliseHeight?"=w419, "Zref"=w418, "Fit Zmax"=w417, "Fit Zmin"=w416, "HeightJitter%"=w415, "Scale"=w411, "BL Targets"=w408, "U,L(U)"=w410, "UtargetsInfo"=w407, "TI,Sigma"=w409, "TItargetsInfo"=w406, "No d0"=w414, "with d0"=w413) -> ("gnuplotOut"=w412:string)  [unwired: 11 in]
          }
        }
        n127 = Select(t="spectraScript", s="Spectra?", f="Write gnuplot file" ("t")) -> (s? t:f=w378:string)
      }
      frame "spectraScript" {
        w447 = 1.0 ("Width")
        w448 = 0.0 ("LateralPosition")
        w454 = 0 ("Active Y Scale")
        n128 = local read "lambda(h)"() -> (w442:dbl)
        n129 = local read "U(h)"() -> (w438:dbl)
        n130 = call "SetSizeAndOriginForMultiplot.vi"("VerticalPosition"=w448, "Height"=w447, "LateralPosition"=w448, "Width"=w447, "ClearLabels?"=TRUE, "PlotLocationDescription"="Bottom plot", "gnuplotIn"=w449) -> ("gnuplotOut"=w444:string)  [unwired: 4 in]
        n131 = Format Into String(format string="$\\\\lambda= %0.2f$m", w442) -> (resulting string=w435:string)  [unwired: 2 in, 1 out]
        n132 = Format Into String(format string="$U(h)= %0.2f$ms$^{-1}$", w438) -> (resulting string=w436:string)  [unwired: 2 in, 1 out]
        n133 = Build Array(w436, w435) -> (w434:string[])
        n134 = control-ref of="Spectrum"() -> (w457:refnum<vi>)
        n135 = call "setLabel.vi"("\"At\" location"=T4 {"XcoordSys"="graph", "YcoordSys"="graph", "Xvalue"=0.98, "Yvalue"=0.85} ("\"At\" location"), "Justify"="right", "multilineLabel"=w434, "String in"=w444) -> ("String out"=w443:string)  [unwired: 6 in, 1 out]
        n136 = call "getAxisBounds.vi"("Active Y Scale"=w454, "Active X Scale"=w454, "XYGraph in"=w457) -> ("Ybounds"=w455:T10, "Xbounds"=w456:T10)  [unwired: 5 in, 2 out]
        n137 = call "AssembleBLMultiplotScript-Spectra.vi"("gnuplotIn"=w443, "SpectrumFilename"=w452, "f.E(f) Bounds"=w455, "f Bounds"=w456) -> ("gnuplotOut"=w453:string)  [unwired: 11 in]
      }
      frame "Write gnuplot file" {
        w479 = FALSE  # append to file? (new file:F)
        w480 = FALSE  # advisory dialog? (display:T)
        n138 = call "chainCommands.vi"("Command"="unset multiplot\t", "Comments"="Close out multiplot", "StringIn"=w467) -> ("StringOut"=w466:string)  [unwired: 8 in]
        n139 = Build Path(base path=w472, name or relative path="gnuplot_script.txt") -> (appended path=w481:path)
        n140 = call "Write_Characters_To_File.vi"("file path (dialog if empty)"=w481, "advisory dialog? (display:T)"=w480, "character string"=w466, "append to file? (new file:F)"=w479) -> ()  [unwired: 1 in, 4 out]
      }
      frame "Execute shell script" {
        n141 = local read "Final Title"() -> (w486:string)
        n142 = Search and Replace String(replace all?=TRUE ("replace all? (F)"), input string=w486, search string=" ", replace string="\\ " ("replace string (\"\")")) -> (result string=w485:string)  [unwired: 4 in, 3 out]
        n143 = Build Path(base path=w488, name or relative path=w485) -> (appended path=w487:path)
        n144 = local read "OutputType"() -> (w483:enum16{"PDF", "PNG-ReportStyle"})
        n145 = call "Run_Gnuplot_Script.vi"("OutputType"=w483, "logfileName"=w496, "workingDirectory"=w487) -> ()
      }
      frame "Has pdf been generated?" {
        n146 = Select(t="Open Standard output file" ("f"), s="OpenLogfile?", f="UI-Monitor" ("t")) -> (s? t:f=w510:string)
        n147 = Select(t="Show Re-Run Gnuplot?", s="Show Script Editor?", f=w510) -> (s? t:f=w513:string)
        n148 = local read "autoprint"() -> (w503:bool)
        n149 = Not(x=w503) -> (.not. x?=w504:bool)
      }
      frame "Show Re-Run Gnuplot?" {
        n150 = local read "OutputType"() -> (w520:enum16{"PDF", "PNG-ReportStyle"})
        n151 = call "Re_run_Gnuplot.vi"("Plot folder (dialog if empty)"=w525, "OutputType"=w520) -> ()  [unwired: 3 out]
      }
      frame "Open Standard output file" {
        n152 = Format Into String(format string="open \"%s\"", w539) -> (resulting string=w538:string)  [unwired: 2 in, 1 out]
        n153 = call <vilib>:"System Exec.vi"("working directory"=w535, "command line"=w538) -> ()  [unwired: 4 in, 6 out]
      }
    }
    "case" <- w24
    "gnuplotScript" <- w21
    "File Path Control" <- w9
  }
  "Saved Automatically?" <- FALSE
